vi "Tree.vi"   [LabVIEW 2016, in "Serial_G.lvlib"]
doc: "TreeVI for viewing all VIs in this driver"
uses:
  Serial_G.lvlib
  Controls/PortConfig.ctl
  Controls/Cmd_Rx.ctl
  Controls/Cmd_Tx.ctl
panel:
  # "VI Tree\nSee Block Diagram"
types:
  T1 = typedef "Serial_G.lvlib/Cmd_Tx.ctl" = cluster{"Write":string, "Fbk?":bool}
  T2 = typedef "Serial_G.lvlib/Cmd_Rx.ctl" = cluster{"Read":string, "ExecTime (ms)":i32, "Timeout?":bool}
  T3 = typedef "Serial_G.lvlib/PortConfig.ctl" = cluster{"Baud rate":u32, "Parity":enum16{"None", "Odd", "Even", "Mark", "Space"}, "Data bits":u16, "Stop bits":u16, "Flow control":u16}
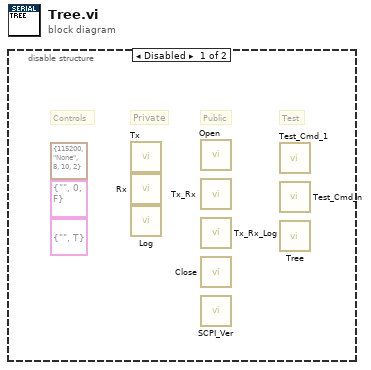
[diagram p0: block diagram]
diagram:
  n1 = disable-structure shown="Disabled" {
    frame Disabled {
      (unwired) T1 {"Write"="", "Fbk?"=TRUE} ("Write")
      (unwired) T2 {"Read"="", "ExecTime (ms)"=0, "Timeout?"=FALSE} ("Read")
      (unwired) T3 {"Baud rate"=115200, "Parity"=enum."None", "Data bits"=8, "Stop bits"=10, "Flow control"=2} ("Cfg Serial Port")
      # "Private"
      # "Test"
      # "Public"
      # "Controls"
      n2 = call "Tx.vi"() -> ()  [unwired: 10 in, 2 out]
      n3 = call "Rx.vi"() -> ()  [unwired: 7 in, 5 out]
      n4 = call "Log.vi"() -> ()  [unwired: 9 in, 3 out]
      n5 = call "Open.vi"() -> ()  [unwired: 8 in, 4 out]
      n6 = call "Tx_Rx.vi"() -> ()  [unwired: 7 in, 5 out]
      n7 = call "Tx_Rx_Log.vi"() -> ()  [unwired: 11 in, 5 out]
      n8 = call "Close.vi"() -> ()  [unwired: 11 in, 1 out]
      n9 = call "SCPI_Ver.vi"() -> ()  [unwired: 7 in, 5 out]
      n10 = call "Test_Cmd_1.vi"() -> ()  [unwired: 10 in, 2 out]
      n11 = call "Test_Cmd_n.vi"() -> ()  [unwired: 11 in, 1 out]
      n12 = call "Tree.vi"() -> ()  [unwired: 16 in]
    }
    frame Enabled {
    }
  }
